vi "Read Attributes.vi"(11 "Instrument Dataset Msg":refnum<class "Instrument Dataset Msg.lvclass">) -> (2 "Payload":T1)   [LabVIEW 2019, in "Instrument.lvlib" / "Instrument Dataset Msg.lvclass"]
uses:
  Instrument Dataset Msg.lvclass
  Instrument Dataset Msg.lvclass/Instrument Dataset Msg.ctl
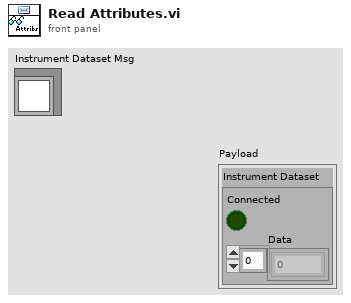
[diagram p1: front panel]
types:
  T1 = cluster{"Instrument Dataset":cluster{"Connected":bool, "Data":dbl[]}}
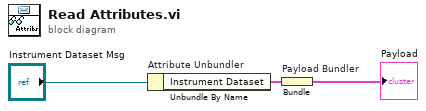
[diagram p0: block diagram]
diagram:
  n1 = Unbundle By Name "Attribute Unbundler"("Instrument Dataset Msg") -> ("Instrument Dataset"=w1:cluster{"Connected":bool, "Data":dbl[]})
  n2 = Bundle "Payload Bundler"("Instrument Dataset"=w1) -> (→"Payload":T1)  [unwired: 1 in]
